vi "主界面.vi"() -> ()   [LabVIEW 2013]
panel:
  in  "reference":refnum<vi>
  in  "调试-界面切换":enum16{"硬件", "项目", "油动机", "采集"}(ring)
  in  "退出":bool
  # "上海电气电站设备有限公司 油动机分析测试软件"
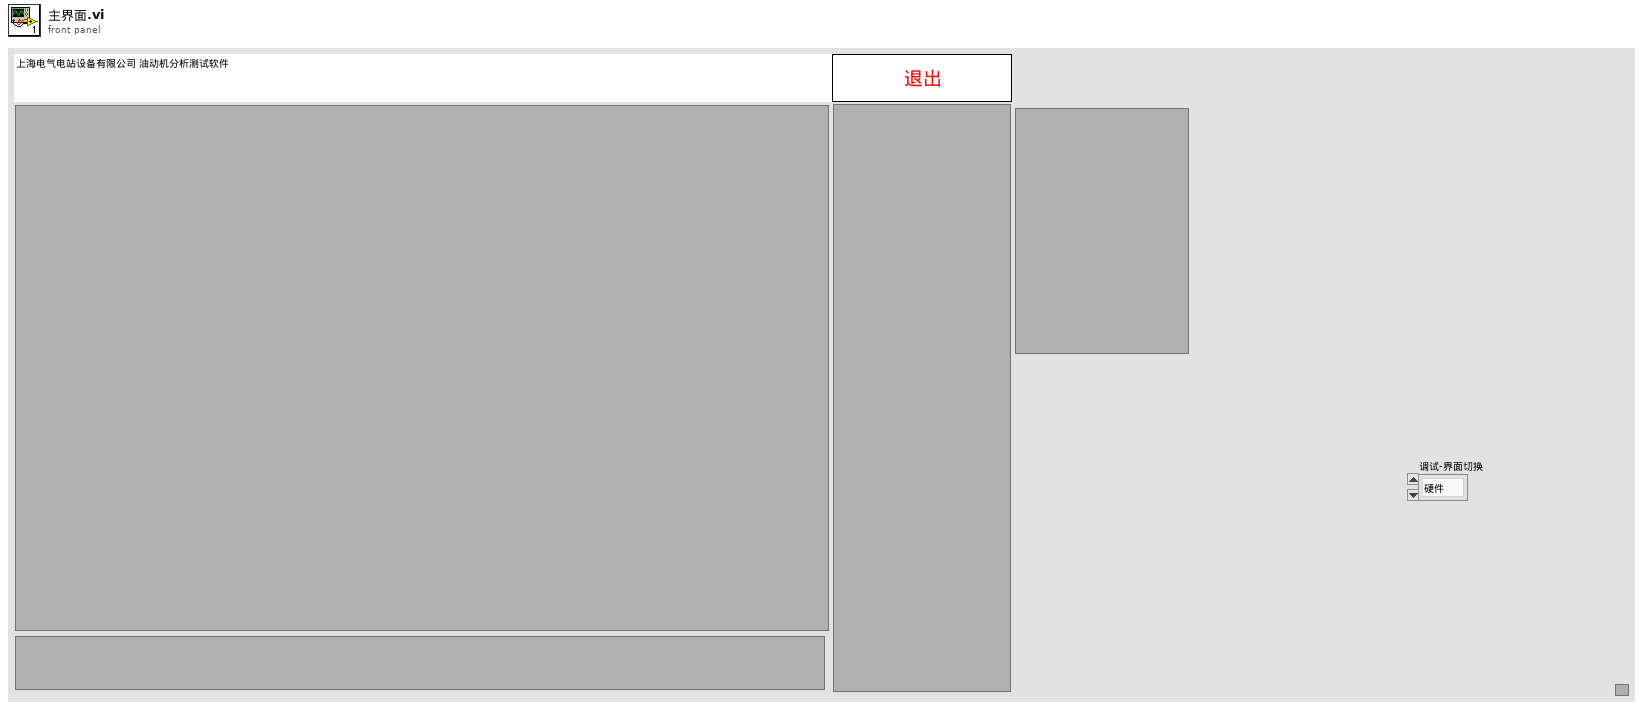
[diagram p1: front panel]
types:
  T1 = enum32{"Bad", "Idle", "Run top level", "Running"}
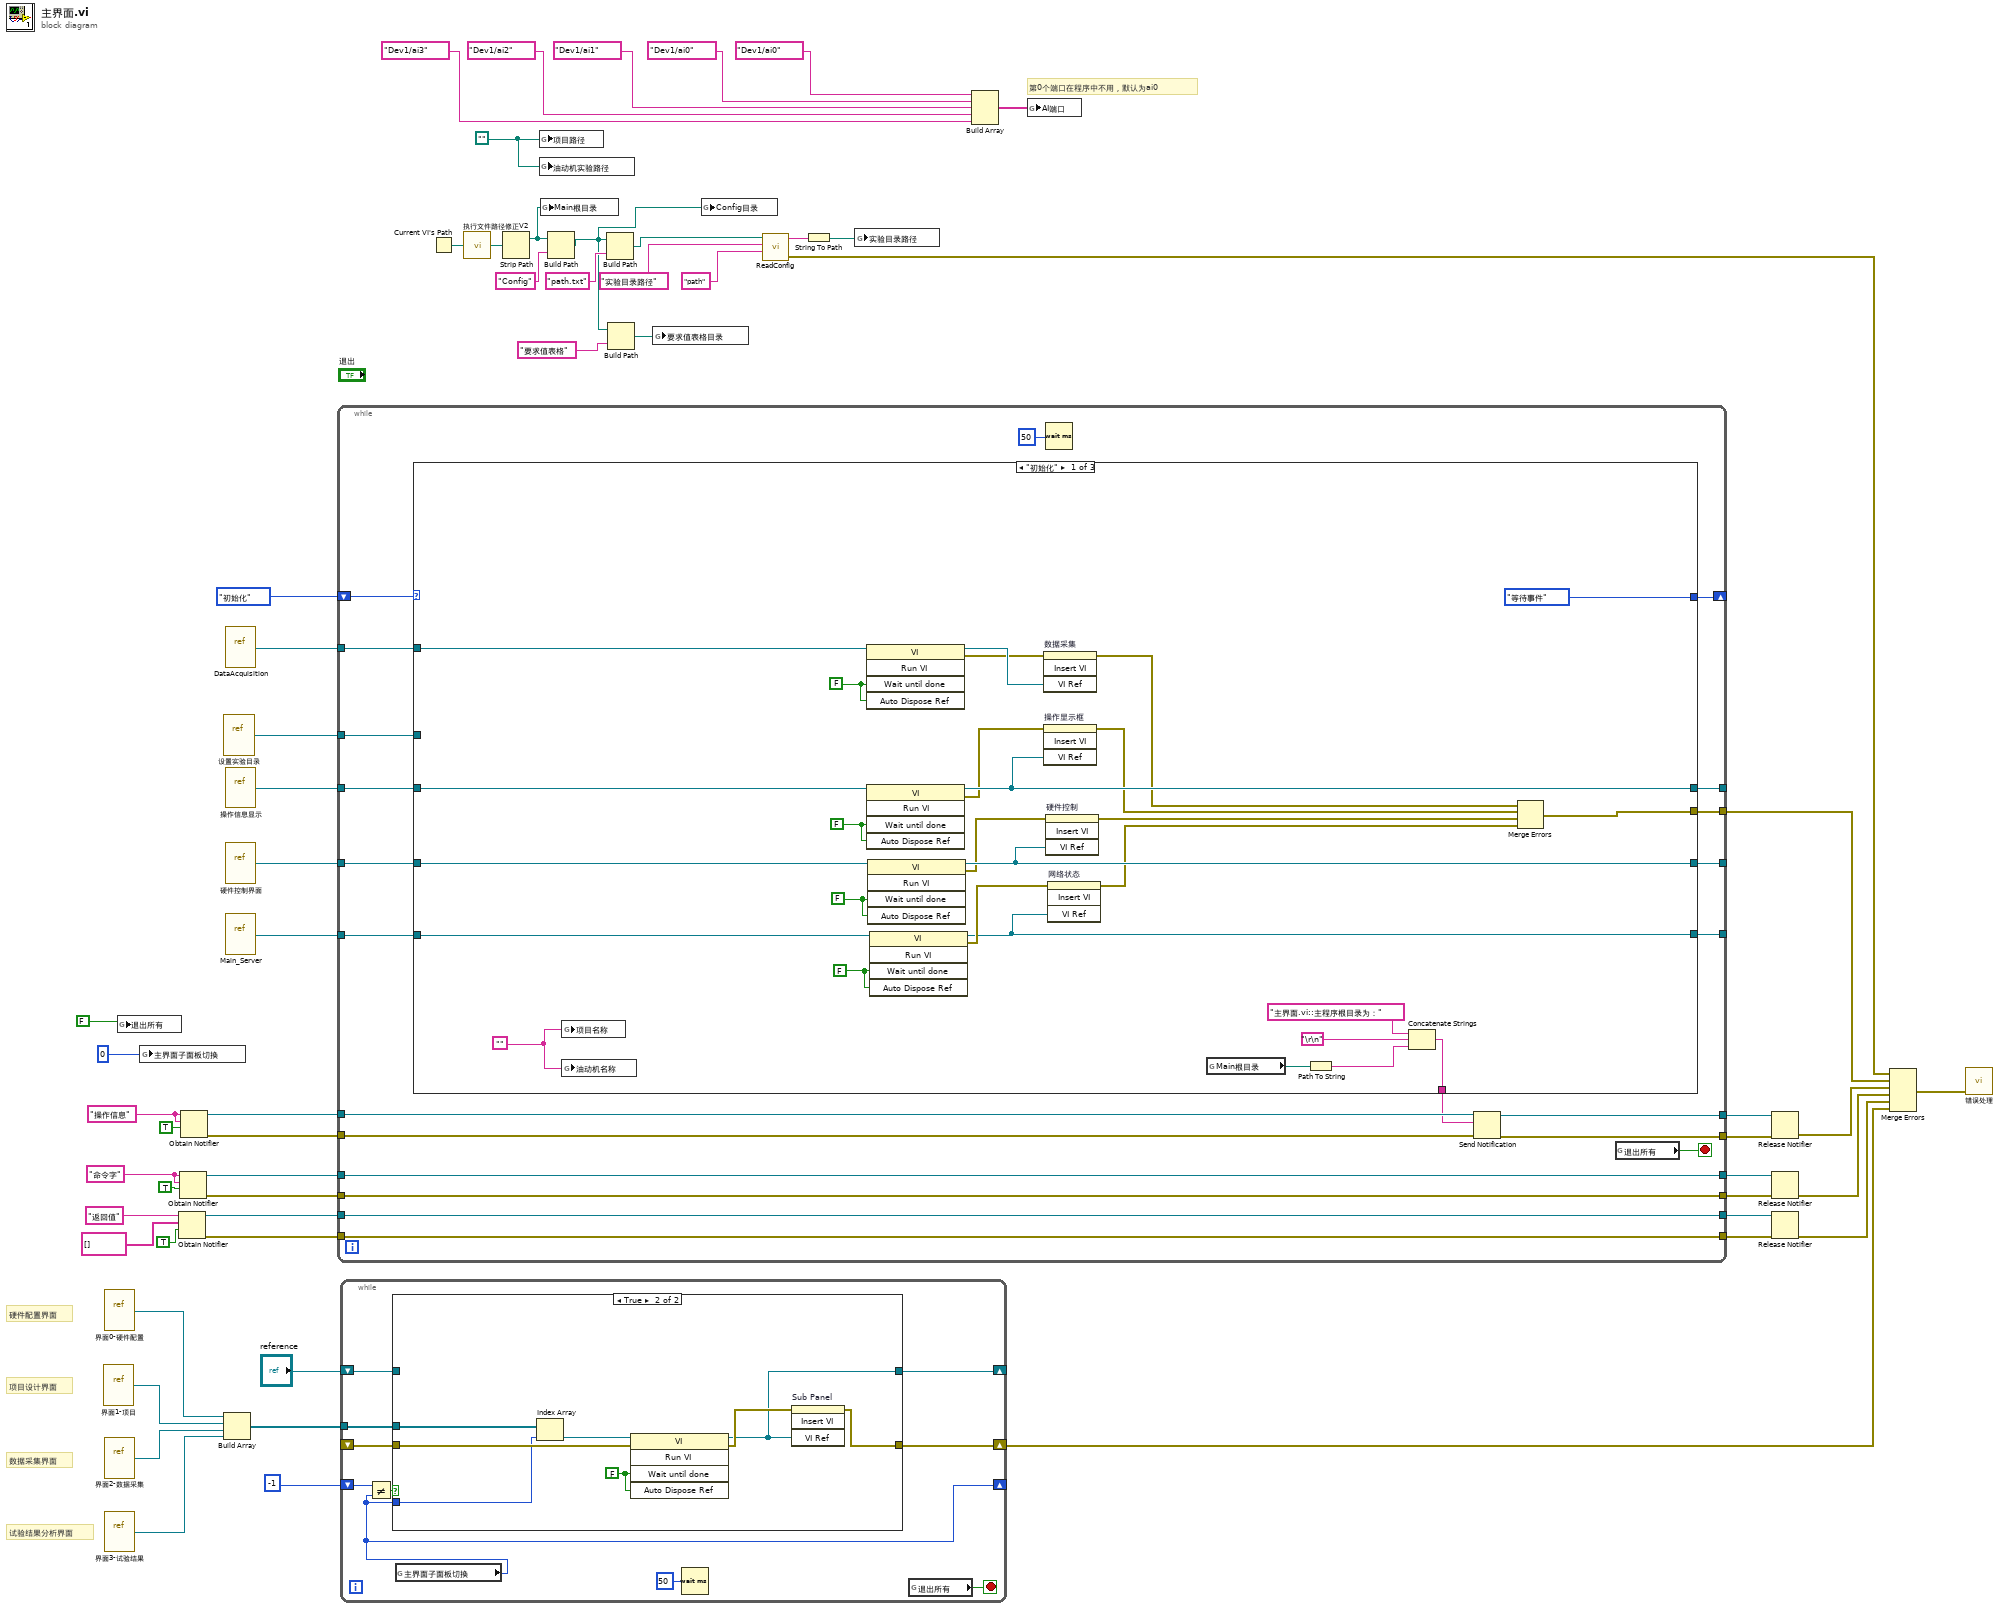
[diagram p0: block diagram]
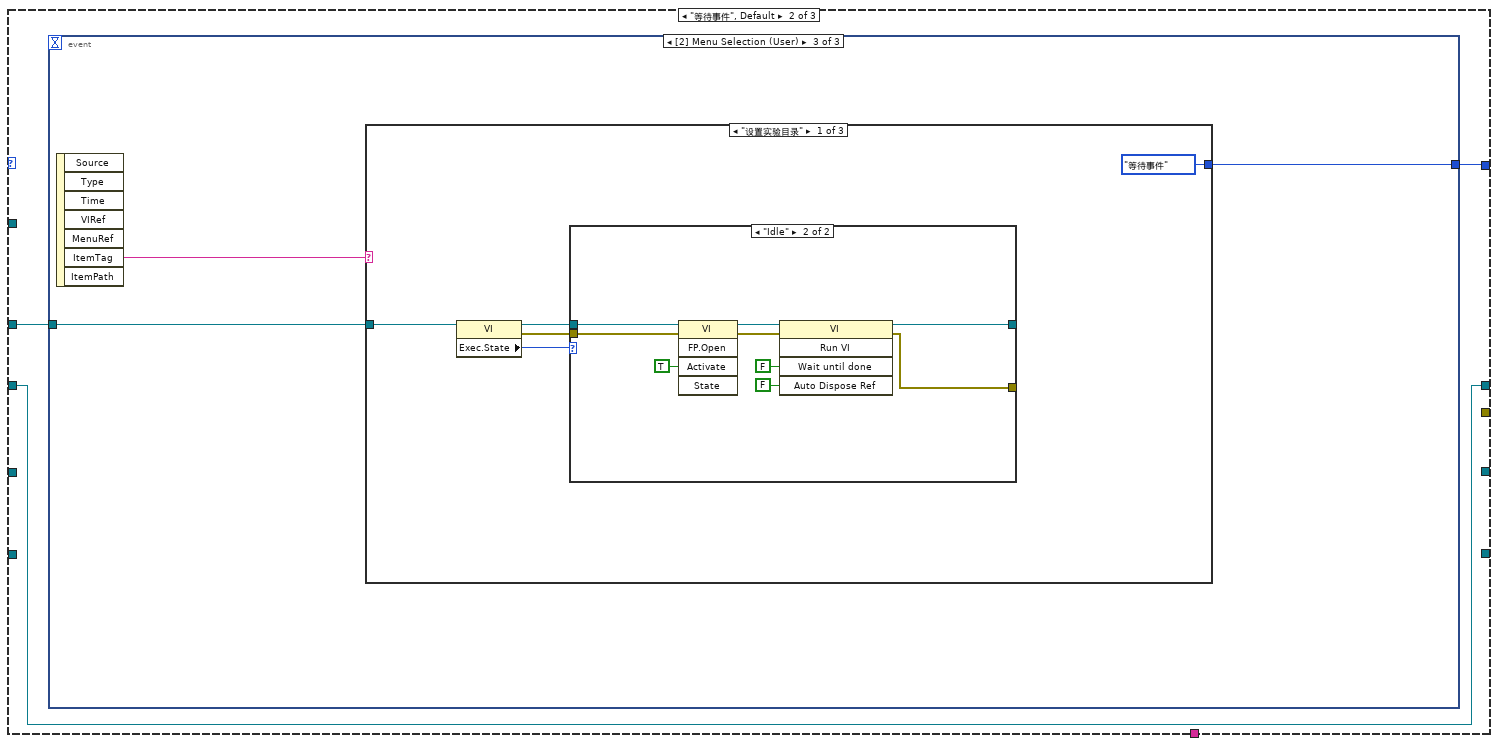
[diagram p3: hidden frame]
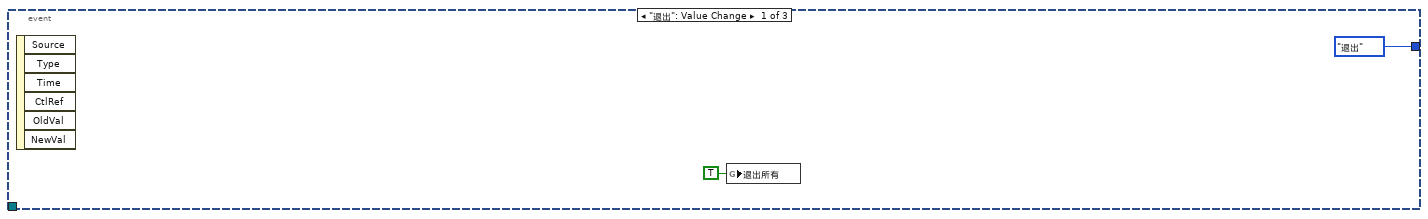
[diagram p4: hidden frame]
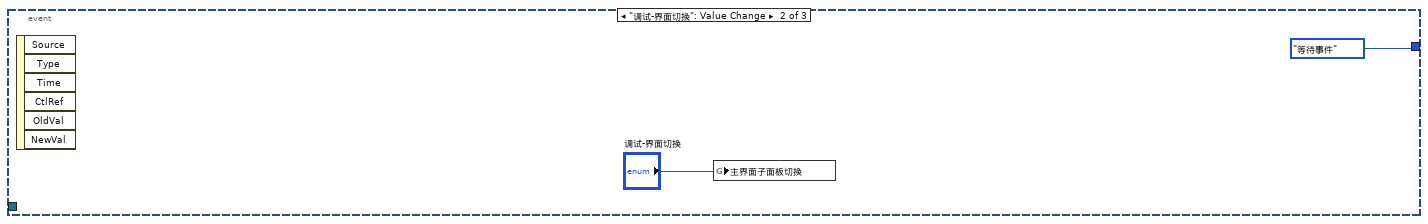
[diagram p5: hidden frame]
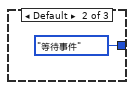
[diagram p7: hidden frame]
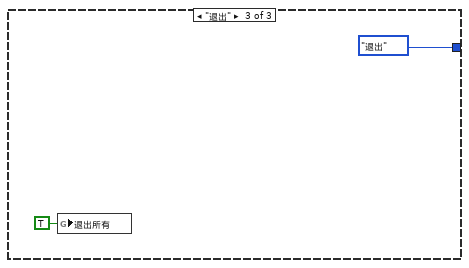
[diagram p8: hidden frame]
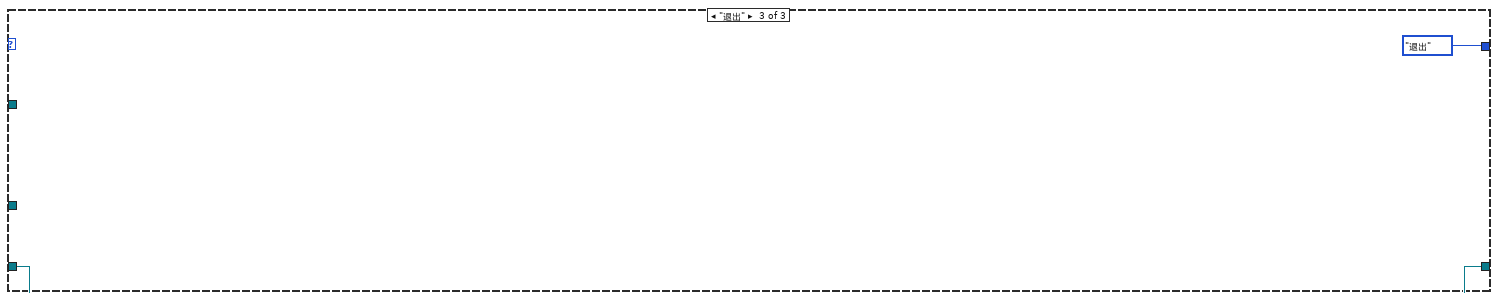
[diagram p9: hidden frame]
diagram:
  w13 = "命令字"
  w40 = path ""
  w60 = "操作信息"
  # "第0个端口在程序中不用，默认为ai0"
  # "试验结果分析界面"
  # "数据采集界面"
  # "项目设计界面"
  # "硬件配置界面"
  n1 = vi-ref "界面1-项目.vi"() -> (w54:refnum<vi>)
  n2 = vi-ref "界面0-硬件配置.vi"() -> (w55:refnum<vi>)
  n3 = vi-ref "界面2-数据采集.vi"() -> (w53:refnum<vi>)
  n4 = vi-ref "界面3-试验结果.vi"() -> (w52:refnum<vi>)
  n5 = global write "退出所有.vi" "退出所有"(FALSE) -> ()
  n6 = global write "主界面子面板切换.vi" "主界面子面板切换"(0) -> ()
  n7 = Obtain Notifier(name (unnamed)="返回值", notification data type=string[] [], create if not found? (T)=TRUE) -> (notifier out=w8:refnum<notifier>, error out=w4:errorcluster)  [unwired: 1 in, 1 out]
  n8 = Obtain Notifier(name (unnamed)=w13, notification data type=w13, create if not found? (T)=TRUE) -> (notifier out=w10:refnum<notifier>, error out=w6:errorcluster)  [unwired: 1 in, 1 out]
  n9 = Obtain Notifier(name (unnamed)=w60, notification data type=w60, create if not found? (T)=TRUE) -> (notifier out=w56:refnum<notifier>, error out=w57:errorcluster)  [unwired: 1 in, 1 out]
  n10 = vi-ref "设置实验目录.vi"() -> (w18:refnum<vi>)
  n11 = Build Array(w55, w54, w53, w52) -> (w50:refnum<vi>[])
  n12 = vi-ref "DataAcquisition.vi"() -> (w25:refnum<vi>)
  n13 = vi-ref "操作信息显示.vi"() -> (w48:refnum<vi>)
  n14 = vi-ref "硬件控制界面.vi"() -> (w39:refnum<vi>)
  n15 = vi-ref "Main_Server.vi"() -> (w17:refnum<vi>)
  n16 = while {
    shift-right: [w82] -> _
    shift-left: enum16{"初始化", "等待事件", "退出"}."初始化" -> [w83]
    tunnel: [w80] -> w59
    tunnel: [w79] -> w58
    tunnel: w57 -> [w78]
    tunnel: w56 -> [w81]
    tunnel: w48 -> [w75]
    tunnel: [w73] -> _
    tunnel: w39 -> [w72]
    tunnel: [w71] -> _
    tunnel: [w70] -> w32
    tunnel: w25 -> [w69]
    tunnel: w18 -> [w68]
    tunnel: w17 -> [w67]
    tunnel: [w66] -> _
    tunnel: [w65] -> w11
    tunnel: w10 -> [w65]
    tunnel: [w64] -> w9
    tunnel: w8 -> [w64]
    tunnel: [w63] -> w7
    tunnel: w6 -> [w63]
    tunnel: [w62] -> w5
    tunnel: w4 -> [w62]
    stop <- w74 stop-if-true
    n17 = case shown="\"初始化\"" w83 {
      tunnel: [enum16{"初始化", "等待事件", "退出"}."等待事件" w114 enum16{"初始化", "等待事件", "退出"}."退出"] -> w82
      tunnel: [w105 _ _] -> w77
      tunnel: w75 -> [w103 w113 w142]
      tunnel: [w102 w113 w142] -> w73
      tunnel: w72 -> [w100 _ _]
      tunnel: [w99 _ _] -> w71
      tunnel: [w94 _ _] -> w70
      tunnel: w69 -> [w92 _ _]
      tunnel: w68 -> [_ w112 _]
      tunnel: w67 -> [w87 _ _]
      tunnel: [w84 _ _] -> w66
      frame "初始化" {
        w88 = FALSE
        w93 = FALSE
        w101 = FALSE
        w104 = FALSE
        w111 = ""
        n18 = global write "项目名称.vi" "项目名称"(w111) -> ()
        n19 = global write "油动机名称.vi" "油动机名称"(w111) -> ()
        n20 = invoke class="VI" method="Run VI"(reference=w92, "Wait until done"=w93, "Auto Dispose Ref"=w93) -> (reference out=w91:refnum<vi>, error out=w89:errorcluster)  [unwired: 2 in, 3 out]
        n21 = invoke class="VI" method="Run VI"(reference=w103, "Wait until done"=w104, "Auto Dispose Ref"=w104) -> (reference out=w102:refnum<vi>, error out=w98:errorcluster)  [unwired: 2 in, 3 out]
        n22 = invoke class="VI" method="Run VI"(reference=w100, "Wait until done"=w101, "Auto Dispose Ref"=w101) -> (reference out=w99:refnum<vi>, error out=w96:errorcluster)  [unwired: 2 in, 3 out]
        n23 = invoke class="VI" method="Run VI"(reference=w87, "Wait until done"=w88, "Auto Dispose Ref"=w88) -> (reference out=w84:refnum<vi>, error out=w86:errorcluster)  [unwired: 2 in, 3 out]
        n24 = invoke on="数据采集" class="SubPnl" method="Insert VI"(error in=w89, "VI Ref"=w91) -> (error out=w90:errorcluster)  [unwired: 2 in, 3 out]
        n25 = invoke on="操作显示框" class="SubPanel" method="Insert VI"(error in=w98, "VI Ref"=w102) -> (error out=w97:errorcluster)  [unwired: 2 in, 3 out]
        n26 = invoke on="硬件控制" class="SubPanel" method="Insert VI"(error in=w96, "VI Ref"=w99) -> (error out=w95:errorcluster)  [unwired: 2 in, 3 out]
        n27 = invoke on="网络状态" class="SubPnl" method="Insert VI"(error in=w86, "VI Ref"=w84) -> (error out=w85:errorcluster)  [unwired: 2 in, 3 out]
        n28 = global read "Main根目录.vi" "Main根目录"() -> (w107:path)
        n29 = Path To String(path=w107) -> (string=w106:string)
        n30 = Concatenate Strings("主界面.vi::主程序根目录为：", "\r\n", w106) -> (w105:string)
        n31 = Merge Errors(w90, w97, w95, w85) -> (w94:errorcluster)
      }
      frame "等待事件", Default {
        n32 = event shown="[2] Menu Selection (User)" {
          selector: _ -> [_ _ _]
          dyn-events: _ -> [_ _ _]
          timeout: _ -> [_ _ _]
          tunnel: [enum16{"初始化", "等待事件", "退出"}."退出" enum16{"初始化", "等待事件", "退出"}."等待事件" w120] -> w114
          tunnel: w112 -> [_ _ w119]
          event "退出": Value Change {
            n33 = event-data() -> ()  [unwired: 1 in, 6 out]
            n34 = global write "退出所有.vi" "退出所有"(TRUE) -> ()
          }
          event "调试-界面切换": Value Change {
            n35 = event-data() -> ()  [unwired: 1 in, 6 out]
            n36 = global write "主界面子面板切换.vi" "主界面子面板切换"("调试-界面切换") -> ()
          }
          event Menu Selection (User) {
            n37 = event-data() -> ("ItemTag"=w121:string)  [unwired: 1 in, 6 out]
            n38 = case shown="\"设置实验目录\"" w121 {
              tunnel: [enum16{"初始化", "等待事件", "退出"}."等待事件" enum16{"初始化", "等待事件", "退出"}."等待事件" enum16{"初始化", "等待事件", "退出"}."退出"] -> w120
              tunnel: w119 -> [w122 _ _]
              frame "设置实验目录" {
                n39 = property class="VI"(reference=w122) -> (reference out=w124:refnum<vi>, error out=w123:errorcluster, "Exec.State"=w125:T1)  [unwired: 1 in]
                n40 = case shown="\"Idle\"" w125 {
                  tunnel: w124 -> [w128 w136]
                  tunnel: [w128 w132] -> _
                  tunnel: w123 -> [w127 w131]
                  tunnel: [w127 w129] -> _
                  frame "Bad", Default {
                  }
                  frame "Idle" {
                    n41 = invoke class="VI" method="FP.Open"(reference=w136, error in=w131, "Activate"=TRUE ("Activate?")) -> (reference out=w134:refnum<vi>, error out=w130:errorcluster)  [unwired: 2 in, 3 out]
                    n42 = invoke class="VI" method="Run VI"(reference=w134, error in=w130, "Wait until done"=FALSE ("Wait Until Done"), "Auto Dispose Ref"=FALSE ("Auto Dispose Reference")) -> (reference out=w132:refnum<vi>, error out=w129:errorcluster)  [unwired: 1 in, 3 out]
                  }
                }
              }
              frame Default {
              }
              frame "退出" {
                n43 = global write "退出所有.vi" "退出所有"(TRUE) -> ()
              }
            }
          }
        }
      }
      frame "退出" {
      }
    }
    n44 = Wait (ms)(milliseconds to wait=50) -> ()  [unwired: 1 out]
    n45 = Send Notification(notification=w77, notifier=w81, error in (no error)=w78) -> (notifier out=w80:refnum<notifier>, error out=w79:errorcluster)
    n46 = global read "退出所有.vi" "退出所有"() -> (w74:bool)
  }
  n47 = while {
    tunnel: w50 -> [w152]
    shift-right: [w150] -> w3
    shift-left: _ -> [w151]
    shift-right: [w144] -> _
    shift-left: -1 -> [w148]
    shift-right: [w146] -> _
    shift-left: "reference" -> [w145]
    stop <- w143 stop-if-true
    n48 = global read "主界面子面板切换.vi" "主界面子面板切换"() -> (w144:i32)
    n49 = Not Equal?(x=w148, y=w144) -> (x != y?=w147:bool)
    n50 = case shown="True" w147 {
      tunnel: w152 -> [_ w162]
      tunnel: w151 -> [w154 w159]
      tunnel: [w154 w157] -> w150
      tunnel: w144 -> [_ w156]
      tunnel: [w153 w155] -> w146
      tunnel: w145 -> [w153 _]
      frame False {
      }
      frame True {
        w160 = FALSE
        n51 = Index Array(array=w162, index=w156) -> (element=w161:refnum<vi>)
        n52 = invoke class="VI" method="Run VI"(reference=w161, error in=w159, "Wait until done"=w160, "Auto Dispose Ref"=w160) -> (reference out=w155:refnum<vi>, error out=w158:errorcluster)  [unwired: 1 in, 3 out]
        n53 = invoke on="Sub Panel" class="SubPnl" method="Insert VI"(error in=w158, "VI Ref"=w155) -> (error out=w157:errorcluster)  [unwired: 2 in, 3 out]
      }
    }
    n54 = Wait (ms)(milliseconds to wait=u32 50) -> ()  [unwired: 1 out]
    n55 = global read "退出所有.vi" "退出所有"() -> (w143:bool)
  }
  n56 = Current VI's Path() -> (path=w28:path)
  n57 = call "执行文件路径修正V2.vi"("Path in"=w28) -> ("Path out"=w27:path)
  n58 = Strip Path(path=w27) -> (stripped path=w26:path)  [unwired: 1 out]
  n59 = global write "项目路径.vi" "项目路径"(w40) -> ()
  n60 = global write "油动机实验路径.vi" "油动机实验路径"(w40) -> ()
  n61 = global write "Main根目录.vi" "Main根目录"(w26) -> ()
  n62 = Build Path(base path=w26, name or relative path="Config") -> (appended path=w36:path)
  n63 = Build Path(base path=w36, name or relative path="path.txt") -> (appended path=w43:path)
  n64 = Build Path(base path=w36, name or relative path="要求值表格") -> (appended path=w38:path)
  n65 = global write "要求值表格目录.vi" "要求值表格目录"(w38) -> ()
  n66 = global write "Config目录.vi" "Config目录"(w36) -> ()
  n67 = call "ReadConfig.vi"("Key"="path", "Section"="实验目录路径", "Path"=w43) -> ("error out"=w30:errorcluster, "Value"=w45:string)  [unwired: 1 in, 1 out]
  n68 = String To Path(string=w45) -> (path=w46:path)
  n69 = global write "实验目录路径.vi" "实验目录路径"(w46) -> ()
  n70 = Build Array(tag "Dev1/ai0" ("电气 2"), tag "Dev1/ai0" ("电气 2"), tag "Dev1/ai1" ("电气"), tag "Dev1/ai2" ("油压"), tag "Dev1/ai3" ("行程")) -> (w19:tag[])
  n71 = global write "AI端口.vi" "AI端口"(w19) -> ()
  n72 = Release Notifier(notifier=w59, error in (no error)=w58) -> (error out=w33:errorcluster)  [unwired: 1 in, 2 out]
  n73 = Release Notifier(notifier=w11, error in (no error)=w7) -> (error out=w2:errorcluster)  [unwired: 1 in, 2 out]
  n74 = Release Notifier(notifier=w9, error in (no error)=w5) -> (error out=w1:errorcluster)  [unwired: 1 in, 2 out]
  n75 = Merge Errors(w30, w32, w33, w2, w1, w3) -> (w31:errorcluster)
  n76 = call "错误处理.vi"("error in (no error)"=w31) -> ()  [unwired: 2 in]
